vi "init j1939.vi"(8 "error in":errorcluster, 10 "stop notifier":refnum<notifier>, 11 "J1939 init data":T1={"CAN Port"="", "CAN Termination"=0, "timing"={"tb to j1939 queue timeout"=100, "j1939 to tb queue timeout"=100, "dtc loop period (ms)"=100, "CAN in loop period (ms)"=100, "process incoming queue timeout (ms)"=100, "Outgoing Write Decimation"=0, "process outgoing loop rate (ms)"=100, "periodic outgoing queue timeout (ms)"=10, "CAN out queue timeout (ms)"=100}, "database"={"BaudRate"=0, "CAN.IoMode"=0, "J1939 Network Address"=0, "Name"=0, "frames"=[]}} {"CAN Termination" items=["Off", "On"]}) -> (0 "error out":errorcluster, 1 "tag bus queues":T6, 2 "data allocations":T26, 3 "J1939 internals":T14={"J1939 XNET Settings"={"XNET Database"="", "XNET Cluster"="", "CAN port"="", "Baud rate [Bd]"=0, "J1939 Network Address"=0, "Name"=0, "Termination"=0}, "j1939 queues"={"Processed Outgoing"=refnum, "Process Outgoing"=refnum, "stop notifier"=refnum, "error queue"=refnum, "active dtc"=refnum, "processed inc"=refnum}, "fgv references"={"BAM Buffer"=refnum, "CM Buffer"=refnum, "CM Gen"=refnum, "BAM Gen"=refnum, "Address Claims"=refnum, "RQST"=refnum, "scaling lut"=refnum, "data lut"=refnum, "cyclic scheduler"=refnum}, "frame in"="", "frame out"="", "timing"={"tb to j1939 queue timeout"=100, "j1939 to tb queue timeout"=100, "dtc loop period (ms)"=100, "CAN in loop period (ms)"=100, "process incoming queue timeout (ms)"=100, "Outgoing Write Decimation"=0, "process outgoing loop rate (ms)"=0, "periodic outgoing queue timeout (ms)"=10, "CAN out queue timeout (ms)"=100}}, 4 "Outgoing Cyclic Cfg":T11 {"Outgoing Cyclic Frame"."Transmit Propreties"."Transmit Time" format="%#_p"}, 5 "Incoming Single Point Configuraiton":T7)   [LabVIEW 2013, in "J1939.lvlib"]
uses:
  J1939.lvlib
  <vilib>/NI/Tag Bus Module Framework/channel/data tables.ctl
  <vilib>/NI/Tag Bus/dictionary/data dictionary.lvclass
  <vilib>/NI/Tag Bus/dictionary table pair.ctl
  <vilib>/NI/Tag Bus/table/data table.ctl
  Internals/API Types/Internal Data.ctl
  Internals/API Types/XNET Settings.ctl
  Users/Benjamin/Desktop/Tag bus J1939/J1939/RT Driver/J1939 Multi Packet Frame/_SubVIs/J1939 Setup Information Cluster.ctl
  Internals/API Types/CAN Outgoing Message Cluster.ctl
  Users/Benjamin/Desktop/Tag bus J1939/J1939/RT Driver/J1939 Multi Packet Frame/_SubVIs/J1939 Convert DTCs Cluster.ctl
  <vilib>/xnet/xnet.llb/XNET Frame CAN.ctl
  <vilib>/xnet/xnet.llb/XNET Frame Type CAN.ctl
  Users/Benjamin/Desktop/Tag bus J1939/J1939/RT Driver/J1939 Multi Packet Frame/_SubVIs/J1939 TP List References.ctl
  Users/Benjamin/Desktop/Tag bus J1939/J1939/RT Driver/J1939 Multi Packet Frame/_SubVIs/J1939 BAM Buffer Connections List_Ref.ctl
  Users/Benjamin/Desktop/Tag bus J1939/J1939/RT Driver/J1939 Multi Packet Frame/_SubVIs/J1939 Connection Mode Generation Connection Ref.ctl
  Users/Benjamin/Desktop/Tag bus J1939/J1939/RT Driver/J1939 Multi Packet Frame/_SubVIs/J1939 BAM Generation Connections List_Ref.ctl
  Internals/LUTs/J1939 Address Table Reference.ctl
  Users/Benjamin/Desktop/Tag bus J1939/J1939/RT Driver/J1939 Multi Packet Frame/_SubVIs/J1939 RQST Lookup Table Reference.ctl
  Internals/LUTs/J1939 Conversion Lookup Table Reference.ctl
  Internals/LUTs/J1939 Data Lookup Table Reference.ctl
  Internals/LUTs/Cyclic Frame Scheduler Lut Reference.ctl
  Configuration/TypeDefs/timing configuration.ctl
  Users/Benjamin/Desktop/Tag bus J1939/J1939/RT Driver/SubVIs/CD Outgoing Cyclic Configuration.ctl
  Users/Benjamin/Desktop/Tag bus J1939/J1939/RT Driver/SubVIs/CD Outgoing Cyclic Frame Pairs.ctl
  Users/Benjamin/Desktop/Tag bus J1939/J1939/RT Driver/SubVIs/XNET Frame Event Properties.ctl
  Internals/API Types/Signal Mapping.ctl
  <vilib>/NI/Tag Bus/tag/Data Type.ctl
  Users/Benjamin/Desktop/Tag bus J1939/J1939/RT Driver/SubVIs/CD Incoming Single Point Configuration.ctl
  Users/Benjamin/Desktop/Tag bus J1939/J1939/RT Driver/SubVIs/CD Incoming Single Point Frame Pairs.ctl
  Internals/API Types/Tag Bus Queues.ctl
  Configuration/TypeDefs/initialization data.ctl
  Configuration/TypeDefs/J1939 db.ctl
  Configuration/TypeDefs/J1939 db frame.ctl
  Configuration/TypeDefs/J1939 db signal.ctl
  Internals/API Types/Scaling Initialization.ctl
  Users/Benjamin/Desktop/Tag bus J1939/J1939/RT Driver/SubVIs/CD Conversion Lookup Table Parameters Cluster.ctl
  <vilib>/NI/Tag Bus Module Framework/channel/TBM channel.lvclass
  <vilib>/NI/Tag Bus/table/data table.lvlib
  <vilib>/NI/Tag Bus/tag bus.lvlib
  <vilib>/NI/Tag Bus/tag/tag descriptor.lvclass
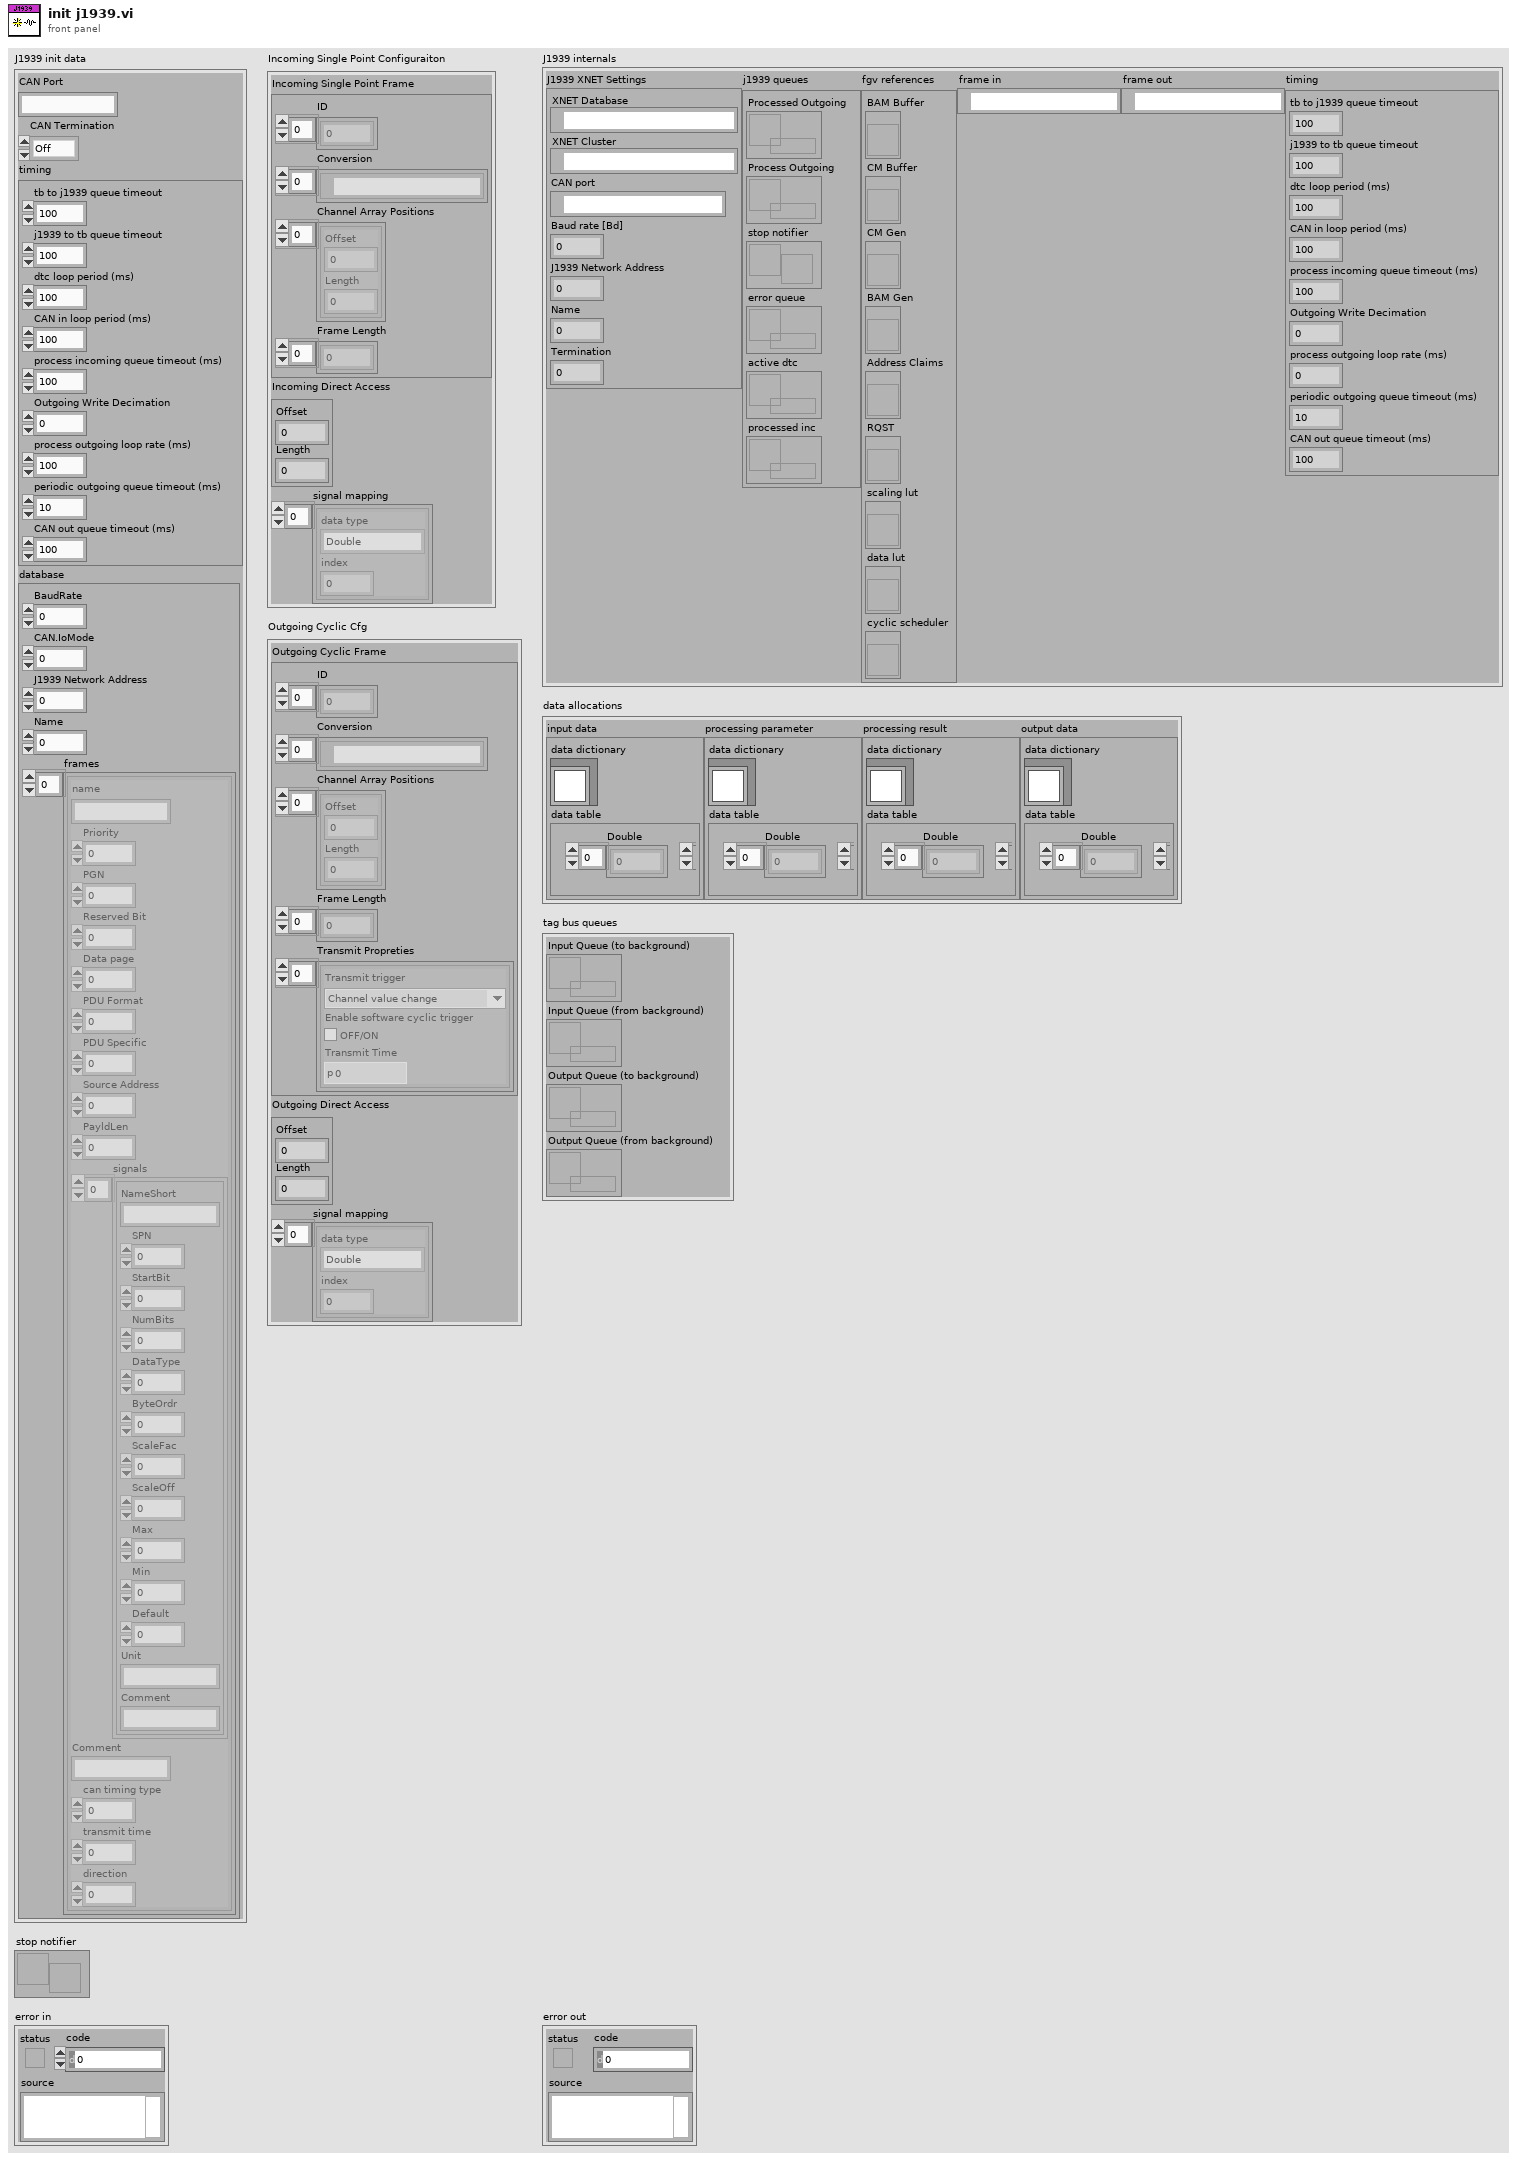
[diagram p1: front panel]
types:
  T1 = typedef "J1939.lvlib/initialization data.ctl" = cluster{"CAN Port":string, "CAN Termination":u32, "timing":T2, "database":T3}
  T2 = typedef "J1939.lvlib/timing configuration.ctl" = cluster{"tb to j1939 queue timeout":i32, "j1939 to tb queue timeout":i32, "dtc loop period (ms)":i32, "CAN in loop period (ms)":i32, "process incoming queue timeout (ms)":i32, "Outgoing Write Decimation":u32, "process outgoing loop rate (ms)":i32, "periodic outgoing queue timeout (ms)":i32, "CAN out queue timeout (ms)":i32}
  T3 = typedef "J1939.lvlib/J1939 db.ctl" = cluster{"BaudRate":u32, "CAN.IoMode":u32, "J1939 Network Address":u8, "Name":u64, "frames":T4[]}
  T4 = typedef "J1939.lvlib/J1939 db frame.ctl" = cluster{"name":string, "Priority":u8, "PGN":u32, "Reserved Bit":u8, "Data page":u8, "PDU Format":u8, "PDU Specific":u8, "Source Address":u8, "PayldLen":u32, "signals":T5[], "Comment":string, "can timing type":u32, "transmit time":dbl, "direction":u16}
  T5 = typedef "J1939.lvlib/J1939 db signal.ctl" = cluster{"NameShort":string, "SPN":i32, "StartBit":u32, "NumBits":u32, "DataType":u32, "ByteOrdr":u32, "ScaleFac":dbl, "ScaleOff":dbl, "Max":dbl, "Min":dbl, "Default":dbl, "Unit":string, "Comment":string}
  T6 = typedef "J1939.lvlib/Tag Bus Queues.ctl" = cluster{"Input Queue (to background)":refnum<queue>, "Input Queue (from background)":refnum<queue>, "Output Queue (to background)":refnum<queue>, "Output Queue (from background)":refnum<queue>}
  T7 = typedef "J1939.lvlib/CD Incoming Single Point Configuration.ctl" = cluster{"Incoming Single Point Frame":T8, "Incoming Direct Access":cluster{"Offset":u32, "Length":u32}, "signal mapping":T9[]}
  T8 = typedef "J1939.lvlib/CD Incoming Single Point Frame Pairs.ctl" = cluster{"ID":u32[], "Conversion":refnum<k21>[], "Channel Array Positions":cluster{"Offset":u32, "Length":u32}[], "Frame Length":u32[]}
  T9 = typedef "J1939.lvlib/signal mapping.ctl" = cluster{"data type":T10, "index":i32}
  T10 = typedef "tag bus.lvlib/tag descriptor.lvclass/Data Type.ctl" = enum16{"Double", "Single", "I64", "I32", "I16", "I8", "U64", "U32", "U16", "U8", "Boolean", "String", "Array of Double", "Array of Single", "Array of I64", "Array of I32", "Array of I16", "Array of I8", "Array of U64", "Array of U32", "Array of U16", "Array of U8", "Array of Boolean", "Array of String"}
  T11 = typedef "J1939.lvlib/CD Outgoing Cyclic Configuration.ctl" = cluster{"Outgoing Cyclic Frame":T12, "Outgoing Direct Access":cluster{"Offset":u32, "Length":u32}, "signal mapping":T9[]}
  T12 = typedef "J1939.lvlib/CD Outgoing Cyclic Frame Pairs.ctl" = cluster{"ID":u32[], "Conversion":refnum<k21>[], "Channel Array Positions":cluster{"Offset":u32, "Length":u32}[], "Frame Length":u32[], "Transmit Propreties":T13[]}
  T13 = typedef "J1939.lvlib/XNET Frame Event Properties.ctl" = cluster{"Transmit trigger":enum16{"Channel value change"}, "Enable software cyclic trigger":bool, "Transmit Time":dbl}
  T14 = typedef "J1939.lvlib/Internal Data.ctl" = cluster{"J1939 XNET Settings":T15, "j1939 queues":T16, "fgv references":T17, "frame in":refnum<k21>, "frame out":refnum<k21>, "timing":T2}
  T15 = typedef "J1939.lvlib/XNET settings.ctl" = cluster{"XNET Database":refnum<k21>, "XNET Cluster":refnum<k21>, "CAN port":refnum<k21>, "Baud rate [Bd]":u32, "J1939 Network Address":u8, "Name":u64, "Termination":u32}
  T16 = typedef "J1939.lvlib/J1939 Setup Information Cluster.ctl" = cluster{"Processed Outgoing":refnum<queue>, "Process Outgoing":refnum<queue>, "stop notifier":refnum<notifier>, "error queue":refnum<queue>, "active dtc":refnum<queue>, "processed inc":refnum<queue>}
  T17 = typedef "J1939.lvlib/J1939 TP List References.ctl" = cluster{"BAM Buffer":T18, "CM Buffer":T18, "CM Gen":T19, "BAM Gen":T20, "Address Claims":T21, "RQST":T22, "scaling lut":T23, "data lut":T24, "cyclic scheduler":T25}
  T18 = typedef "J1939.lvlib/J1939 BAM Buffer Connections List_Ref.ctl" = refnum<vi>
  T19 = typedef "J1939.lvlib/J1939 Connection Mode Generation Connection Ref.ctl" = refnum<vi>
  T20 = typedef "J1939.lvlib/J1939 BAM Generation Connections List_Ref.ctl" = refnum<vi>
  T21 = typedef "J1939.lvlib/J1939 Address Table Reference.ctl" = refnum<vi>
  T22 = typedef "J1939.lvlib/J1939 RQST Lookup Table Reference.ctl" = refnum<vi>
  T23 = typedef "J1939.lvlib/J1939 Conversion Lookup Table Reference.ctl" = refnum<vi>
  T24 = typedef "J1939.lvlib/J1939 Data Lookup Table Reference.ctl" = refnum<vi>
  T25 = typedef "J1939.lvlib/cyclic frame scheduler lut reference.ctl" = refnum<vi>
  T26 = typedef "TBM channel.lvclass/data tables.ctl" = cluster{"input data":T27, "processing parameter":T27, "processing result":T27, "output data":T27}
  T27 = typedef "tag bus.lvlib/dictionary table pair.ctl" = cluster{"data dictionary":refnum<class "data dictionary.lvclass">, "data table":T28}
  T28 = typedef "tag bus.lvlib/data table.lvlib/data table.ctl" = cluster{"Double":dbl[], "Single":sgl[], "I64":i64[], "I32":i32[], "I16":i16[], "I8":i8[], "U64":u64[], "U32":u32[], "U16":u16[], "U8":u8[], "Boolean":bool[], "String":string[], "Array of Double":cluster{"DBL Array":dbl[]}[], "Array of Single":cluster{"SGL Array":sgl[]}[], "Array of I64":cluster{"I64 Array":i64[]}[], "Array of I32":cluster{"I32 Array":i32[]}[], "Array of I16":cluster{"I16 Array":i16[]}[], "Array of I8":cluster{"I8 Array":i8[]}[], "Array of U64":cluster{"U64 Array":u64[]}[], "Array of U32":cluster{"U32 Array":u32[]}[], "Array of U16":cluster{"U16 Array":u16[]}[], "Array of U8":cluster{"U8 Array":u8[]}[], "Array of Boolean":cluster{"Boolean Array":bool[]}[], "Array of String":cluster{"String Array":string[]}[]}
  T29 = typedef "J1939.lvlib/scaling initialization.ctl" = cluster{"input names":string[], "inputs":T30[], "output names":string[], "outputs":T30[]}
  T30 = typedef "J1939.lvlib/CD Conversion Lookup Table Parameters Cluster.ctl" = cluster{"Conversion":refnum<k21>, "Array Position":cluster{"Offset":u32, "Length":u32}, "Length":u32, "Conv ID":u32}
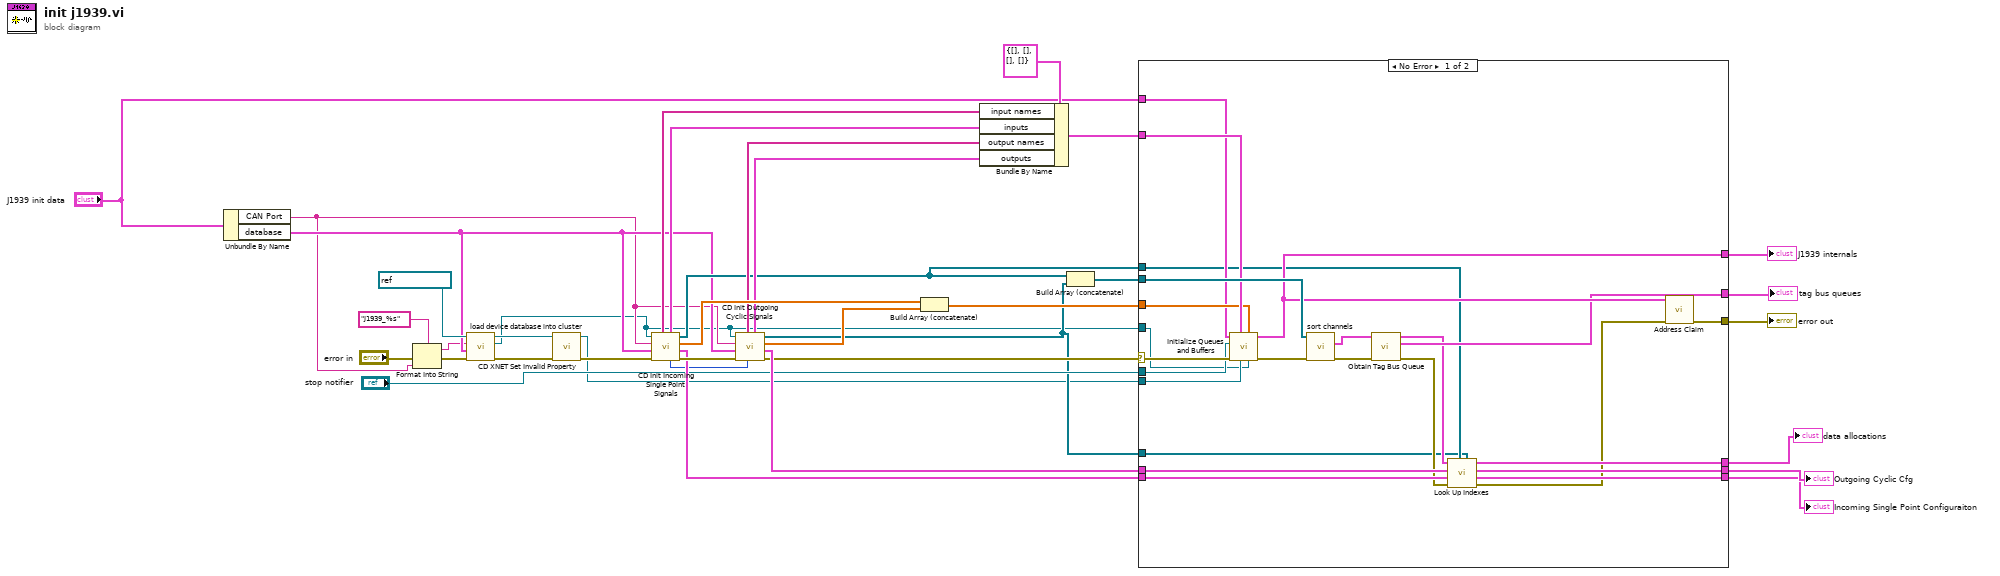
[diagram p0: block diagram]
diagram:
  n1 = Unbundle By Name("J1939 init data") -> ("CAN Port"=w5:string, "database"=w8:T3)
  n2 = Format Into String(format string="J1939_%s", error in="error in", w5) -> (resulting string=w4:string, error out=w6:errorcluster)  [unwired: 1 in]
  n3 = call "load device database into cluster.vi"("error in"=w6, "system db"=w8, "cluster name (CAN0)"=w4, "database in"=refnum<k21> ":memory:") -> ("error out"=w10:errorcluster, "cluster out"=w1:refnum<k21>, "database out"=w7:refnum<k21>)  [unwired: 5 in]
  n4 = call "CD XNET Set Invalid Property.vi"("error in"=w10, "XNET Database"=w7) -> ("error out"=w37:errorcluster, "database out"=w2:refnum<k21>)  [unwired: 8 in]
  n5 = call "CD Init Incoming Single Point Signals.vi"("error in"=w37, "database"=w8, "can port"=w5, "XNET Cluster"=w1) -> ("error out"=w36:errorcluster, "Incoming Single Point Configuraiton"=w21:T7, "initial value"=w29:dbl[], "channels"=w14:refnum<class "TBM channel.lvclass">[], "# of Channels"=w12:u32, "inputs"=w28:T30[], "input IDs"=w27:string[])  [unwired: 1 in]
  n6 = call "CD Init Outgoing Cyclic Signals.vi"("Memory Table Offset"=w12, "error in"=w36, "database"=w8, "can port"=w5, "XNET Cluster"=w1) -> ("error out"=w17:errorcluster, "Outgoing Cyclic Configuraiton"=w19:T11, "initial values"=w26:dbl[], "channels"=w13:refnum<class "TBM channel.lvclass">[], "outputs"=w24:T30[], "output IDs"=w25:string[])  [unwired: 1 in]
  n7 = Build Array (concatenate)(w29, w26) -> (w32:dbl[])
  n8 = Bundle By Name(cluster=T29 {"input names"=[], "inputs"=[], "output names"=[], "outputs"=[]}, "input names"=w27, "inputs"=w28, "output names"=w25, "outputs"=w24) -> (w33:T29)
  n9 = Build Array (concatenate)(w14, w13) -> (w35:refnum<class "TBM channel.lvclass">[])
  n10 = case shown="No Error" w17 {
    selector: w17 -> [w44 w64]
    tunnel: w35 -> [w60 _]
    tunnel: w33 -> [w59 _]
    tunnel: w32 -> [w58 _]
    tunnel: [w57 w64] -> w31
    tunnel: [w56 _] -> w30
    tunnel: [w55 w63] -> w23
    tunnel: [w54 w62] -> w22
    tunnel: w21 -> [w53 w62]
    tunnel: [w52 _] -> w20
    tunnel: w19 -> [w50 w63]
    tunnel: [w46 _] -> w18
    tunnel: "stop notifier" -> [w43 _]
    tunnel: "J1939 init data" -> [w42 _]
    tunnel: w14 -> [w41 _]
    tunnel: w13 -> [w40 _]
    tunnel: w2 -> [w39 _]
    tunnel: w1 -> [w38 _]
    frame No Error {
      n11 = call "Initialize Queues and Buffers.vi"("XNET Cluster"=w38, "initial values"=w58, "XNET Database"=w39, "scaling information"=w59, "error in"=w44, "stop notifier"=w43, "J1939 init data"=w42) -> ("error out"=w61:errorcluster, "j1939 internals"=w56:T14)  [unwired: 3 in]
      n12 = call <vilib>:"sort channels.vi"("error in"=w61, "channels in"=w60) -> ("error out"=w49:errorcluster, "data allocations"=w47:T26)  [unwired: 7 in, 1 out]
      n13 = call "Obtain Tag Bus Queue.vi"("error in"=w49, "data allocations"=w47) -> ("error out"=w48:errorcluster, "tag bus queues"=w46:T6, "data allocations out"=w45:T26)  [unwired: 7 in]
      n14 = call "Look Up Indexes.vi"("outgoing channels"=w40, "incoming channels"=w41, "error in"=w48, "Incoming Single Point Configuraiton in"=w53, "Outgoing Cyclic Configuration in"=w50, "data allocations in"=w45) -> ("error out"=w51:errorcluster, "Incoming Single Point Configuraiton out"=w54:T7, "Outgoing Cyclic Configuration out"=w55:T11, "data allocations out"=w52:T26)  [unwired: 2 in]
      n15 = call "Address Claim.vi"("error in"=w51, "J1939 Internals"=w56) -> ("error out"=w57:errorcluster)  [unwired: 9 in]
    }
    frame Error {
    }
  }
  "error out" <- w31
  "J1939 internals" <- w30
  "Outgoing Cyclic Cfg" <- w23
  "Incoming Single Point Configuraiton" <- w22
  "data allocations" <- w20
  "tag bus queues" <- w18
